vi "Hella CAN Turbine.vi"(8 "Error IN":errorcluster, 11 "CMD":u8) -> (0 "Error OUT":errorcluster)   [LabVIEW 2013]
uses:
  Type Defs/CAN Mode.ctl
  <vilib>/RioEmbeddedCAN/RioEmbeddedCAN.llb/CANFrameControl.ctl
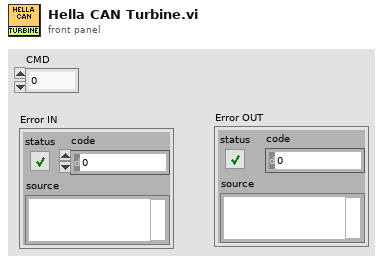
[diagram p1: front panel]
types:
  T1 = typedef "CAN Mode.ctl" = enum16{"Init", "Read", "Write", "Close"}
  T2 = typedef "CANFrameControl.ctl" = cluster{"identifier":u32, "extended?":bool, "type":enum8{"CAN Data", "CAN Remote"}, "payload":u8[]}
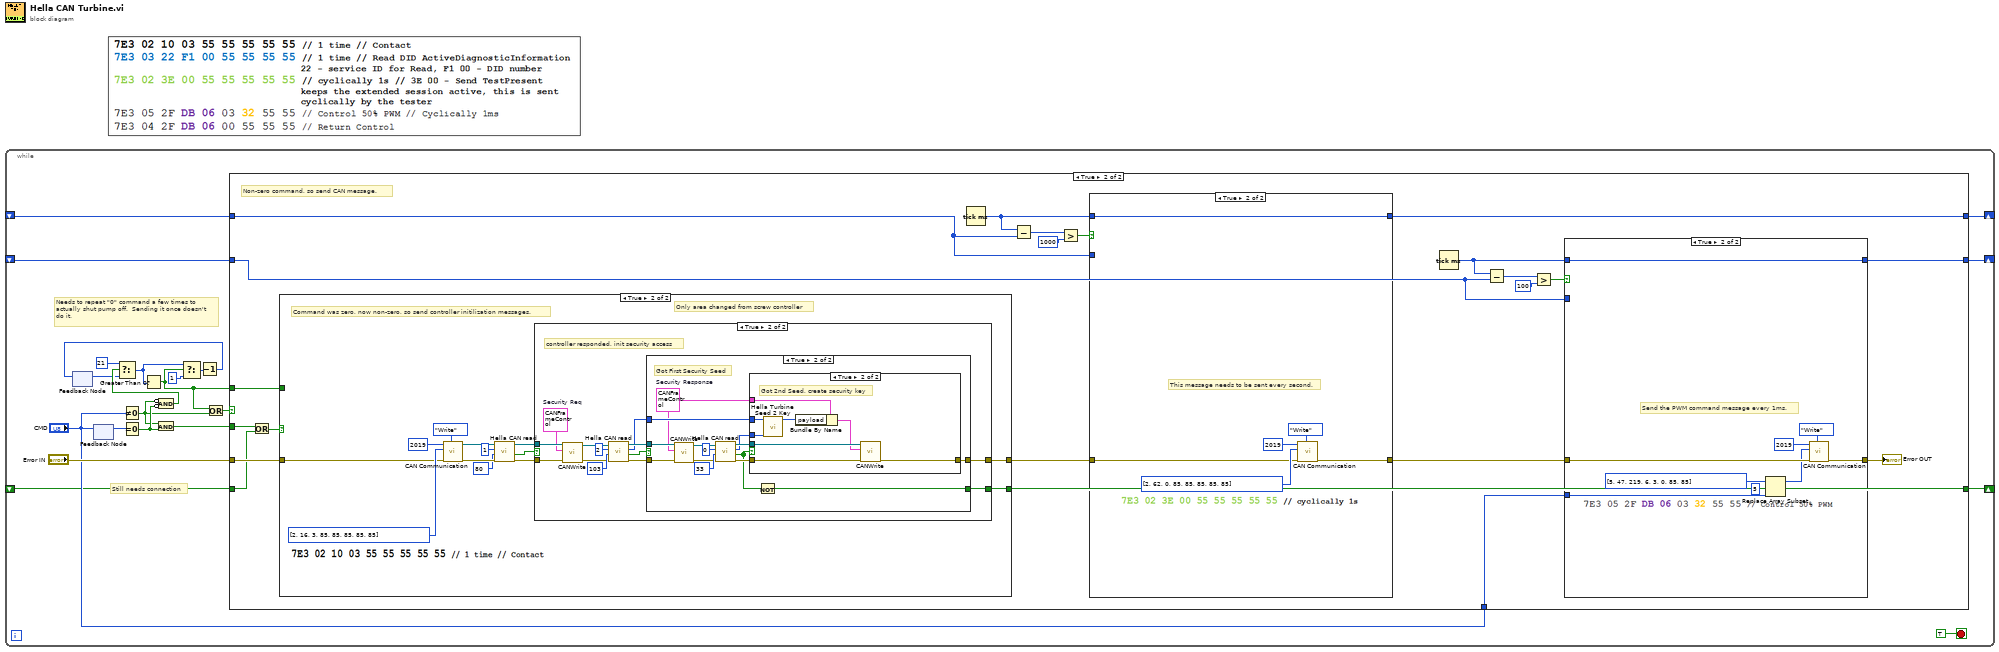
[diagram p0: block diagram]
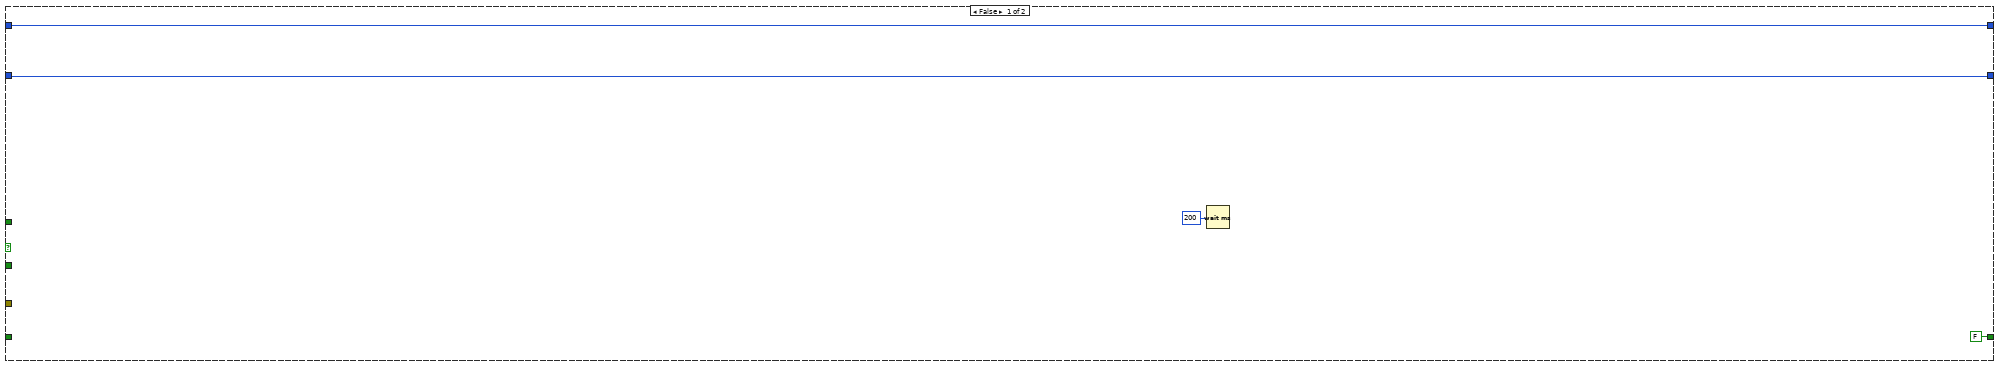
[diagram p2: hidden frame]
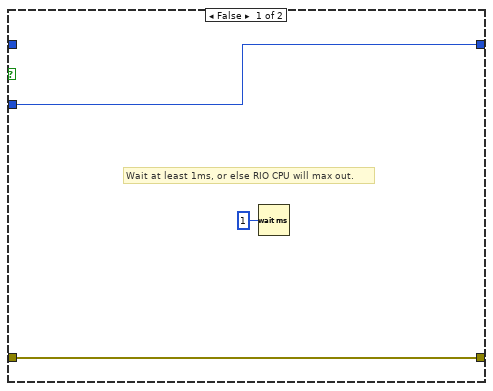
[diagram p3: hidden frame]
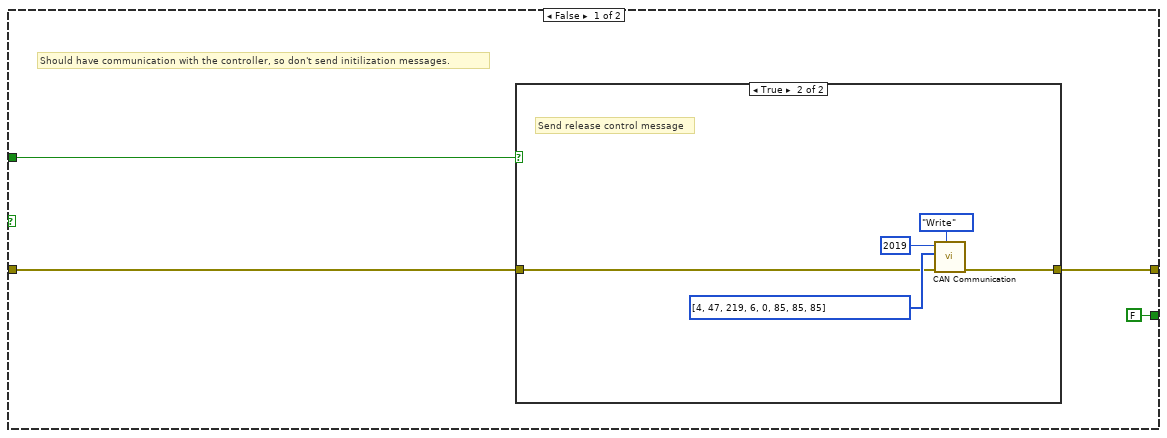
[diagram p5: hidden frame]
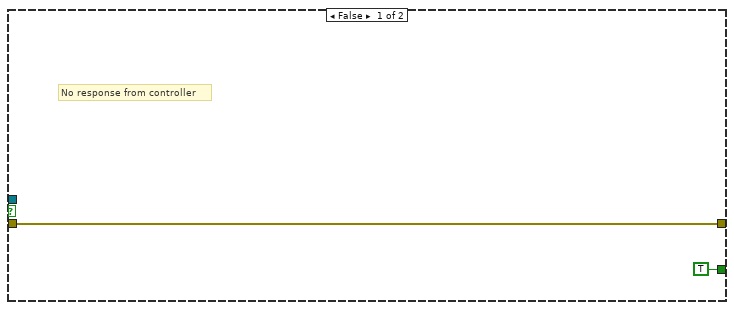
[diagram p7: hidden frame]
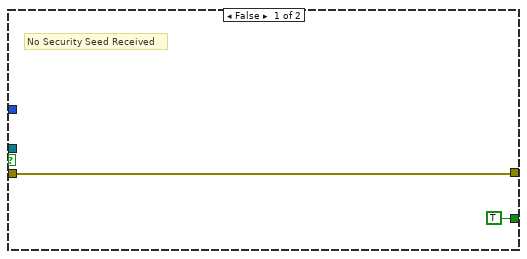
[diagram p8: hidden frame]
diagram:
  n1 = while {
    shift-right: [w19] -> _
    shift-left: _ -> [w18]
    shift-right: [w17] -> _
    shift-left: _ -> [w16]
    shift-right: [w3] -> _
    shift-left: _ -> [w2]
    stop <- TRUE stop-if-true
    # "Still needs connection"
    # "Needs to repeat \"0\" command a few times to\nactually shut pump off.  Sending it once doesn't\ndo it."
    n2 = feedback #1() -> (w10:i32)  [unwired: 1 in]
    n3 = feedback #2() -> (w22:u8)  [unwired: 1 in]
    n4 = feedback-in #2("CMD") -> ()
    n5 = Not Equal To 0?(x="CMD") -> (x != 0?=w5:bool)
    n6 = Equal To 0?(x=w22) -> (x = 0?=w6:bool)
    n7 = And(x=w5, y=w6) -> (x .and. y?=w4:bool)
    n8 = Compound Arithmetic op=AND(invert w5, invert w6) -> (w12:bool)
    n9 = Select(t=21, s=w12, f=w10) -> (s? t:f=w9:i32)
    n10 = Greater Than 0?(x=w9) -> (x > 0?=w1:bool)
    n11 = Select(t=w9, s=w1, f=1) -> (s? t:f=w8:i32)
    n12 = Decrement(x=w8) -> (x-1=w11:i32)
    n13 = feedback-in #1(w11) -> ()
    n14 = Or(x=w1, y=w5) -> (x .or. y?=w14:bool)
    n15 = case shown="True" w14 {
      tunnel: w4 -> [_ w30]
      tunnel: "Error IN" -> [_ w48]
      tunnel: [w26 w42] -> w19
      tunnel: w18 -> [w26 w41]
      tunnel: [w25 w37] -> w17
      tunnel: w16 -> [w25 w35]
      tunnel: "CMD" -> [_ w33]
      tunnel: [FALSE w31] -> w3
      tunnel: w2 -> [_ w28]
      tunnel: w1 -> [_ w27]
      frame False {
        n16 = Wait (ms)(milliseconds to wait=u32 200) -> ()  [unwired: 1 out]
      }
      frame True {
        # "Non-zero command, so send CAN message."
        n17 = Or(x=w30, y=w28) -> (x .or. y?=w29:bool)
        n18 = case shown="True" w29 {
          tunnel: w48 -> [w70 w88]
          tunnel: [w69 w81] -> w47
          tunnel: [FALSE w79] -> w31
          tunnel: w27 -> [w71 _]
          frame False {
            # "Should have communication with the controller, so don't send initilization messages."
            n19 = case shown="True" w71 {
              tunnel: w70 -> [w73 w75]
              tunnel: [w73 w74] -> w69
              frame False {
                # "Running, do nothing here"
              }
              frame True {
                # "Send release control message"
                n20 = call "CAN Communication.vi"("CAN Mode"=CAN_Mode."Write", "Error IN"=w75, "Message"=u8[] [4, 47, 219, 6, 0, 85, 85, 85] ("array"), "Arbitration ID"=u32 2019 ("CAN Addres to Xmit\nSpeed CMD (Hex) 2")) -> ("Error OUT"=w74:errorcluster)  [unwired: 6 in, 1 out]
              }
            }
          }
          frame True {
            # "Only area changed from screw controller"
            # "Command was zero, now non-zero, so send controller initilization messages."
            n21 = call "CAN Communication.vi"("CAN Mode"=CAN_Mode."Write", "Error IN"=w88, "Message"=u8[] [2, 16, 3, 85, 85, 85, 85, 85] ("array"), "Arbitration ID"=u32 2019 ("CAN Addres to Xmit\nSpeed CMD (Hex) 2")) -> ("Error OUT"=w86:errorcluster, "CAN Ref"=w87:refnum<k20>)  [unwired: 6 in]
            n22 = call "Hella CAN read.vi"("Error In"=w86, "Expected"=u8 80, "Index"=1, "Ref In"=w87) -> ("Error Out"=w84:errorcluster, "Valid?"=w80:bool, "Ref Out"=w85:refnum<k20>)  [unwired: 4 in, 1 out]
            n23 = case shown="True" w80 {
              tunnel: w85 -> [_ w106]
              tunnel: w84 -> [w93 w105]
              tunnel: [w93 w98] -> w81
              tunnel: [TRUE w94] -> w79
              frame False {
                # "No response from controller"
              }
              frame True {
                w97 = T2 {"identifier"=2019, "extended?"=FALSE, "type"=enum."CAN Data", "payload"=[2, 39, 55, 0, 0, 0, 0, 0]}  # Security Req
                # "controller responded, init security access"
                n24 = call <vilib>:"CANWrite.vi"("error in (no error)"=w105, "CAN frame"=w97, "interface object in"=w106) -> ("error out"=w99:errorcluster, "interface object out"=w102:refnum<k20>)  [unwired: 7 in]
                n25 = call "Hella CAN read.vi"("Error In"=w99, "Expected"=u8 103, "Index"=2, "Ref In"=w102) -> ("Error Out"=w100:errorcluster, "Valid?"=w96:bool, "payload"=w95:u8[], "Ref Out"=w101:refnum<k20>)  [unwired: 4 in]
                n26 = case shown="True" w96 {
                  tunnel: w101 -> [_ w120]
                  tunnel: w100 -> [w108 w119]
                  tunnel: [w108 w114] -> w98
                  tunnel: w95 -> [_ w112]
                  tunnel: [TRUE w109] -> w94
                  frame False {
                    # "No Security Seed Received"
                  }
                  frame True {
                    w111 = T2 {"identifier"=2019, "extended?"=FALSE, "type"=enum."CAN Data", "payload"=[48, 8, 0, 0, 0, 0, 0, 0]}  # Security Response
                    # "Got First Security Seed"
                    n27 = call <vilib>:"CANWrite.vi"("error in (no error)"=w119, "CAN frame"=w111, "interface object in"=w120) -> ("error out"=w117:errorcluster, "interface object out"=w118:refnum<k20>)  [unwired: 7 in]
                    n28 = call "Hella CAN read.vi"("Error In"=w117, "Expected"=u8 33, "Index"=0, "Ref In"=w118) -> ("Error Out"=w116:errorcluster, "Valid?"=w110:bool, "payload"=w113:u8[], "Ref Out"=w115:refnum<k20>)  [unwired: 4 in]
                    n29 = case shown="True" w110 {
                      tunnel: w116 -> [w123 w131]
                      tunnel: w115 -> [_ w130]
                      tunnel: [w123 w129] -> w114
                      tunnel: w113 -> [_ w128]
                      tunnel: w112 -> [_ w127]
                      tunnel: w111 -> [_ w126]
                      frame False {
                        # "Did not get second security seed"
                      }
                      frame True {
                        # "Got 2nd Seed, create security key"
                        n30 = call "Hella Turbine Seed 2 Key.vi"("MSG 2"=w128, "MSG 1"=w127) -> ("Security Response"=w125:u8[])  [unwired: 9 in]
                        n31 = Bundle By Name(cluster=w126, "payload"=w125) -> (w124:T2)
                        n32 = call <vilib>:"CANWrite.vi"("error in (no error)"=w131, "CAN frame"=w124, "interface object in"=w130) -> ("error out"=w129:errorcluster)  [unwired: 7 in, 1 out]
                      }
                    }
                    n33 = Not(x=w110) -> (.not. x?=w109:bool)
                  }
                }
              }
            }
          }
        }
        n34 = Tick Count (ms)() -> (millisecond timer value=w43:u32)
        n35 = Subtract(x=w43, y=w41) -> (x-y=w46:u32)
        n36 = Greater?(x=w46, y=u32 1000) -> (0:w44:bool)
        n37 = case shown="True" w44 {
          tunnel: w47 -> [w61 w65]
          tunnel: [w62 w64] -> w42
          tunnel: w43 -> [_ w64]
          tunnel: w41 -> [w62 _]
          tunnel: [w61 w63] -> w34
          frame False {
          }
          frame True {
            # "This message needs to be sent every second."
            n38 = call "CAN Communication.vi"("CAN Mode"=CAN_Mode."Write", "Error IN"=w65, "Message"=u8[] [2, 62, 0, 85, 85, 85, 85, 85] ("array"), "Arbitration ID"=u32 2019 ("CAN Addres to Xmit\nSpeed CMD (Hex) 2")) -> ("Error OUT"=w63:errorcluster)  [unwired: 6 in, 1 out]
          }
        }
        n39 = Tick Count (ms)() -> (millisecond timer value=w38:u32)
        n40 = Subtract(x=w38, y=w35) -> (x-y=w39:u32)
        n41 = Greater?(x=w39, y=u32 100) -> (0:w36:bool)
        n42 = case shown="True" w36 {
          tunnel: w34 -> [w50 w58]
          tunnel: [w50 w57] -> w32
          tunnel: [w51 w56] -> w37
          tunnel: w38 -> [_ w56]
          tunnel: w35 -> [w51 _]
          tunnel: w33 -> [_ w52]
          frame False {
            # "Wait at least 1ms, or else RIO CPU will max out."
            n43 = Wait (ms)(milliseconds to wait=u32 1) -> ()  [unwired: 1 out]
          }
          frame True {
            # "Send the PWM command message every 1ms."
            n44 = Replace Array Subset(array=u8[] [5, 47, 219, 6, 3, 0, 85, 85], new element=w52, index=5) -> (w53:u8[])
            n45 = call "CAN Communication.vi"("CAN Mode"=CAN_Mode."Write", "Error IN"=w58, "Message"=w53, "Arbitration ID"=u32 2019 ("CAN Addres to Xmit\nSpeed CMD (Hex) 2")) -> ("Error OUT"=w57:errorcluster)  [unwired: 6 in, 1 out]
          }
        }
        "Error OUT" <- w32
      }
    }
  }
